vi "Wait-for-message.vi"(8 "error in (no error)":errorcluster, 11 "Client in":T1) -> (0 "error out":errorcluster, 1 "New message?":bool, 2 "Message":refnum<class "Message.lvclass">, 3 "Client out":T1)   [LabVIEW 2013, in "PowderDeposition.lvlib" / "PD-Client.lvclass"]
doc: "Monitors the incomming communication channel (client channel) for new messages.\nThe monitoring will timeout based on the 'Heartbeat interval' parameter in the client settings. The timeout time is 80% of the heartbeat interval value, to allow the client to send a heartbeat message and have it processed by the server. The heartbeat is separate functionality, acessed through the 'Send-heartbeat' function."
uses:
  PD-Client.lvclass
  Object-reference.ctl
  SA-SLMAPI/Sources/Message.lvclass
  PD-Client.lvclass/PD-Client.ctl
  Read Client channel.vi
  Read Heartbeat interval.vi
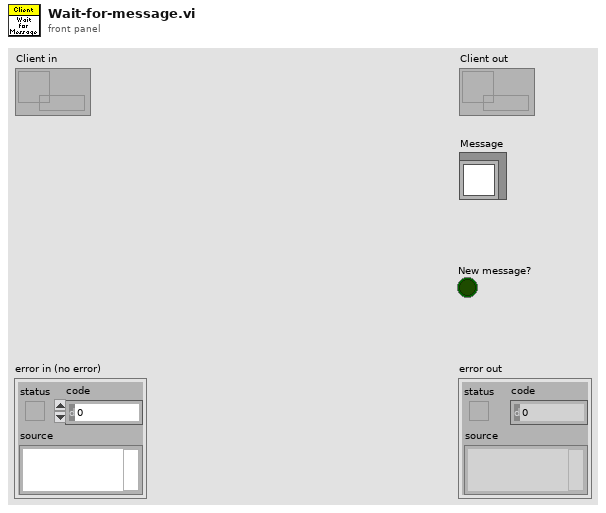
[diagram p1: front panel]
types:
  T1 = typedef "PowderDeposition.lvlib/PD-Client.lvclass/Object-reference.ctl" = refnum<data-value>
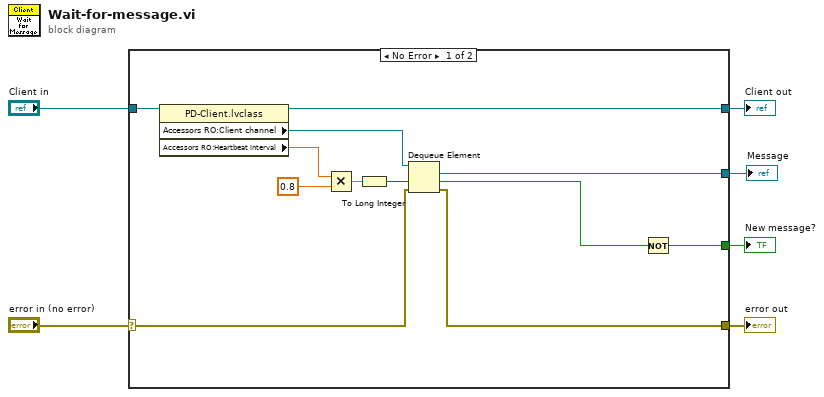
[diagram p0: block diagram]
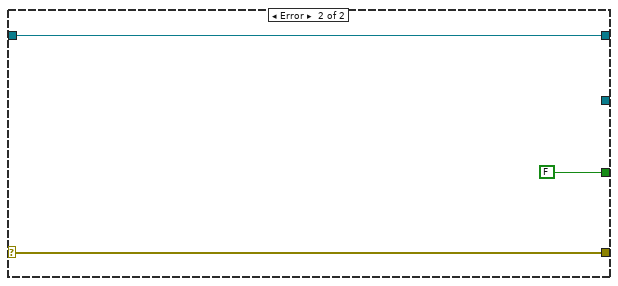
[diagram p2: hidden frame]
diagram:
  n1 = case shown="No Error" "error in (no error)" {
    selector: "error in (no error)" -> [w8 w21]
    tunnel: [w7 w21] -> w5
    tunnel: [w17 w20] -> w3
    tunnel: "Client in" -> [w18 w20]
    tunnel: [w13 FALSE ("New?")] -> w2
    tunnel: [w14 _] -> w1
    frame No Error {
      n2 = property class="PD-Client.lvclass"(reference=w18) -> (reference out=w17:T1, "Accessors RO:Client channel"=w16:refnum<queue>, "Accessors RO:Heartbeat interval"=w12:dbl)  [unwired: 1 in, 1 out]
      n3 = Multiply(x=w12, y=0.8) -> (x*y=w11:dbl)
      n4 = To Long Integer(number=w11) -> (32bit integer=w9:i32)
      n5 = Dequeue Element(queue=w16, timeout in ms (-1)=w9, error in (no error)=w8) -> (element=w14:refnum<class "Message.lvclass">, timed out?=w15:bool, error out=w7:errorcluster)  [unwired: 1 out]
      n6 = Not(x=w15) -> (.not. x?=w13:bool)
    }
    frame Error {
    }
  }
  "error out" <- w5
  "Client out" <- w3
  "New message?" <- w2
  "Message" <- w1
